vi "Jiggle standalone.vi"(0 "GEA2 Reference In":refnum<k24>, 2 "Standalone?":bool, 5 "GEA Inputs":T1={"Source"=228, "Destination"=35} {"Destination" format="%.0x"; "Source" format="%.0x"}, 7 "Modeshift To":enum16{"Agitate", "Spin"}(ring), 9 "Timeout (s)":dbl=60.0 format="%0.2f", 11 "Error In":errorcluster) -> (4 "GEA2 Reference Out":refnum<k24>, 6 "Pass/Fail?":bool, 8 "Report Text":string, 15 "Error Out":errorcluster)   [LabVIEW 2016, in "TLMB.lvlib"]
uses:
  Projects/TLMB.lvlib
  Common/LabVIEW GEA2 Toolkit/LabVIEW_GEA2_Toolkit.lvlibp/type defs/Source_Destination.ctl
  Q:/Common/DLLs/GEA3/GeaCommunication.dll
  Common/DLLs/GEA3/GeaCommunication.dll
  Common/LabVIEW GEA2 Toolkit/LabVIEW_GEA2_Toolkit.lvlibp/type defs/ERD Write Data In.ctl
  Common/LabVIEW GEA2 Toolkit/LabVIEW_GEA2_Toolkit.lvlibp/type defs/Data Type.ctl
  <vilib>/DAQmx/read.llb/DAQmx Read (Digital 1D Wfm NChan NSamp).vi
  <vilib>/DAQmx/create/channels.llb/DAQmx Create Channel (DI-Digital Input).vi
  <vilib>/DAQmx/configure/timing.llb/DAQmx Timing (Sample Clock).vi
  <vilib>/DAQmx/configure/trigger.llb/DAQmx Start Trigger (Digital Edge).vi
  <vilib>/DAQmx/miscellaneous.llb/DAQmx Fill In Error Info.vi
  Common/LabVIEW GEA2 Toolkit/LabVIEW_GEA2_Toolkit.lvlibp
panel:
  out "Results":dbl[][](array[numeric])=[[0.0, 0.1, 0.9, 0.1], [1.5, 0.0, 0.0, 0.0]]
  in  "Lower Limits":dbl[][](array[numeric])=[[0.0, 0.05, 0.85, 0.05], [1.45, 0.0, 0.0, 0.0]]
  in  "Upper Limits":dbl[][](array[numeric])=[[0.0, 0.15, 0.95, 0.15], [1.55, 0.0, 0.0, 0.0]]
  out "Digital Waveform Graph":digitalwaveform[](graph)
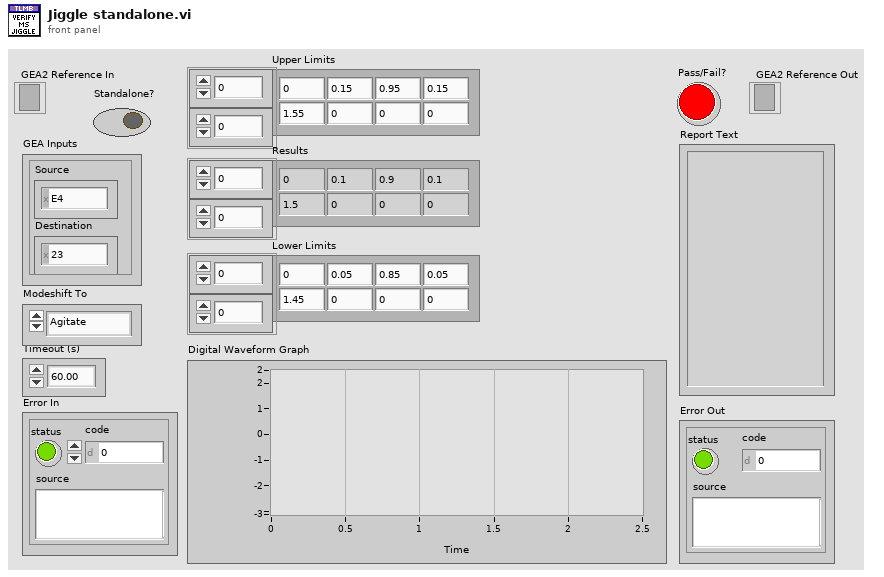
[diagram p1: front panel]
types:
  T1 = typedef "LabVIEW_GEA2_Toolkit.lvlibp/Source_Destination.ctl" = cluster{"Source":u8, "Destination":u8}
  T2 = typedef "LabVIEW_GEA2_Toolkit.lvlibp/ERD Write Data In.ctl" = cluster{"ERD Number":u16, "Data Type":T3, "Data":string}
  T3 = typedef "LabVIEW_GEA2_Toolkit.lvlibp/Data Type.ctl" = enum16{"string", "boolean", "uint8_t", "uint16_t", "uint32_t", "uint64_t", "int8_t", "int16_t", "int32_t", "int64_t"}
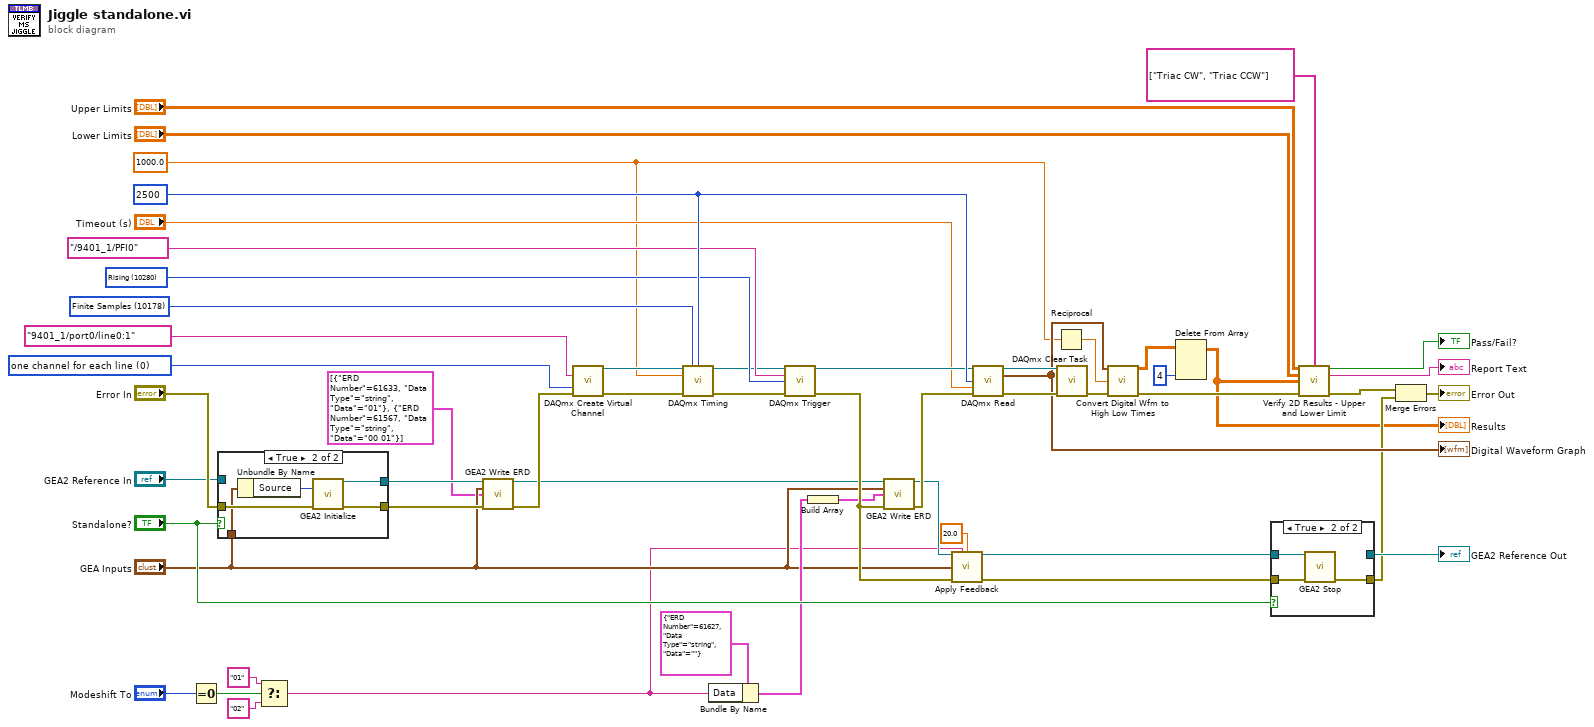
[diagram p0: block diagram]
diagram:
  w45 = 10280 items=["Rising"=10280, "Falling"=10171] ("edge")
  w50 = 0 items=["one channel for each line", "one channel for all lines"] ("line grouping")
  w38 = 1000.0 ("rate")
  w47 = 2500 ("samples per channel")
  w52 = 10178 items=["Finite Samples"=10178, "Continuous Samples"=10123, "Hardware Timed Single Point"=12522] ("sample mode")
  n1 = Equal To 0?(x="Modeshift To") -> (x = 0?=w13:bool)
  n2 = case shown="True" "Standalone?" {
    tunnel: [w56 w61] -> w12
    tunnel: "Error In" -> [w56 w60]
    tunnel: [w55 w59] -> w9
    tunnel: "GEA2 Reference In" -> [w55 _]
    tunnel: "GEA Inputs" -> [_ w58]
    frame False {
    }
    frame True {
      n3 = Unbundle By Name(w58) -> ("Source"=w57:u8)
      n4 = call "GEA2 Initialize.vi"("Source Address"=w57, "error in"=w60) -> ("GEA2 Reference Out"=w59:refnum<k24>, "error out"=w61:errorcluster)  [unwired: 11 in, 1 out]
    }
  }
  n5 = Select(t="01", s=w13, f="02") -> (s? t:f=w6:string)
  n6 = call "GEA2 Write ERD.vi"("GEA2 Reference In"=w9, "GEA Inputs"="GEA Inputs", "Write ERD List"=T2[] [{"ERD Number"=61633, "Data Type"=enum."string", "Data"="01"}, {"ERD Number"=61567, "Data Type"=enum."string", "Data"="00 01"}], "Error In"=w12) -> ("GEA2 Reference Out"=w10:refnum<k24>, "Error Out"=w11:errorcluster)  [unwired: 9 in, 1 out]
  n7 = call-poly <vilib>:"DAQmx Create Virtual Channel.vi"("lines"=tag "9401_1/port0/line0:1", "line grouping"=w50, "error in"=w11) -> ("task out"=w54:refnum<k21>, "error out"=w53:errorcluster)  [unwired: 11 in]
  n8 = call-poly <vilib>:"DAQmx Timing.vi"("task/channels in"=w54, "sample mode"=w52, "samples per channel"=w47, "rate"=w38, "error in"=w53) -> ("task out"=w44:refnum<k21>, "error out"=w42:errorcluster)  [unwired: 9 in]
  n9 = Bundle By Name(cluster=T2 {"ERD Number"=61627, "Data Type"=enum."string", "Data"=""} ("ERD Write Data In"), "Data"=w6) -> (w15:T2)
  n10 = call-poly <vilib>:"DAQmx Trigger.vi"("task/channels in"=w44, "source"=tag "/9401_1/PFI0", "edge"=w45, "error in"=w42) -> ("task out"=w43:refnum<k21>, "error out"=w27:errorcluster)  [unwired: 10 in]
  n11 = Build Array(w15) -> (w17:T2[])
  n12 = call "GEA2 Write ERD.vi"("GEA2 Reference In"=w10, "GEA Inputs"="GEA Inputs", "Write ERD List"=w17, "Error In"=w27) -> ("GEA2 Reference Out"=w25:refnum<k24>, "Error Out"=w26:errorcluster)  [unwired: 9 in, 1 out]
  n13 = call "Apply Feedback.vi"("GEA2 Reference In"=w25, "Expected Modeshift Mode"=w6, "Timeout (s)"=20.0, "GEA Inputs"="GEA Inputs", "Error In"=w27) -> ("GEA2 Reference Out"=w29:refnum<k24>, "Error Out"=w24:errorcluster)  [unwired: 9 in]
  n14 = call-poly <vilib>:"DAQmx Read.vi"("task/channels in"=w43, "number of samples per channel"=w47, "timeout"="Timeout (s)", "error in"=w26) -> ("task out"=w49:refnum<k21>, "data"=w40:digitalwaveform[], "error out"=w48:errorcluster)  [unwired: 9 in]
  "Digital Waveform Graph" <- w40
  n15 = Reciprocal(x=w38) -> (1/x=w39:dbl)
  n16 = call <vilib>:"DAQmx Clear Task.vi"("task in"=w49, "error in"=w48) -> ("error out"=w37:errorcluster)  [unwired: 13 in]
  n17 = call "Convert Digital Wfm to High Low Times.vi"("Digital Waveform In"=w40, "Dt"=w39, "Error In"=w37) -> ("HL Raw Output"=w33:dbl[][], "Error Out"=w36:errorcluster)  [unwired: 11 in]
  n18 = Delete From Array(array=w33, index (col)=4 ("disabled index (col)")) -> (array with subset deleted=w1:dbl[][])  [unwired: 2 in, 1 out]
  "Results" <- w1
  n19 = case shown="True" "Standalone?" {
    tunnel: w29 -> [w63 w66]
    tunnel: w24 -> [w62 w65]
    tunnel: [w62 w64] -> w18
    tunnel: [w63 _] -> w21
    frame False {
    }
    frame True {
      n20 = call "GEA2 Stop.vi"("GEA2 Reference In"=w66, "Error In"=w65) -> ("Error Out"=w64:errorcluster)  [unwired: 13 in]
    }
  }
  "GEA2 Reference Out" <- w21
  n21 = call "Verify 2D Results - Upper and Lower Limit.vi"("Upper Limits"="Upper Limits", "Array of Names"=string[] ["Triac CW", "Triac CCW"], "Lower Limits"="Lower Limits", "Results"=w1, "Error In"=w36) -> ("Pass/Fail?"=→"Pass/Fail?":bool, "Report Text"=→"Report Text":string, "Error Out"=w19:errorcluster)  [unwired: 7 in, 1 out]
  n22 = Merge Errors(w19, w18) -> (→"Error Out":errorcluster)
